vi "test_SetItemInfoDependencies.vi"() -> (3 "Pass?":bool)   [LabVIEW 2020, in "Tests.SolutionBuilder.lvlib"]
uses:
  Tests.SolutionBuilder.lvlib
  SolutionBuilder/SolutionBuilder.lvclass
  SolutionBuilder/ProjectItem/ProjectItem.lvclass
panel:
  out "test results":u32 format="%02b"
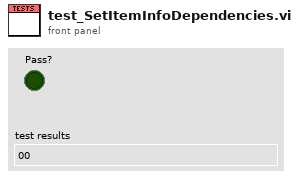
[diagram p1: front panel]
types:
  T1 = cluster{"Relative Path from 1 to 2":path, string[]}[]
  T2 = typedef "SolutionBuilder.lvlib/SolutionBuilder.lvclass/ProjectItemMap.ctl" = map{path, refnum<class "ProjectItem.lvclass">[]}
  T3 = cluster{"Relative Path from 1 to 2":path, string[]}
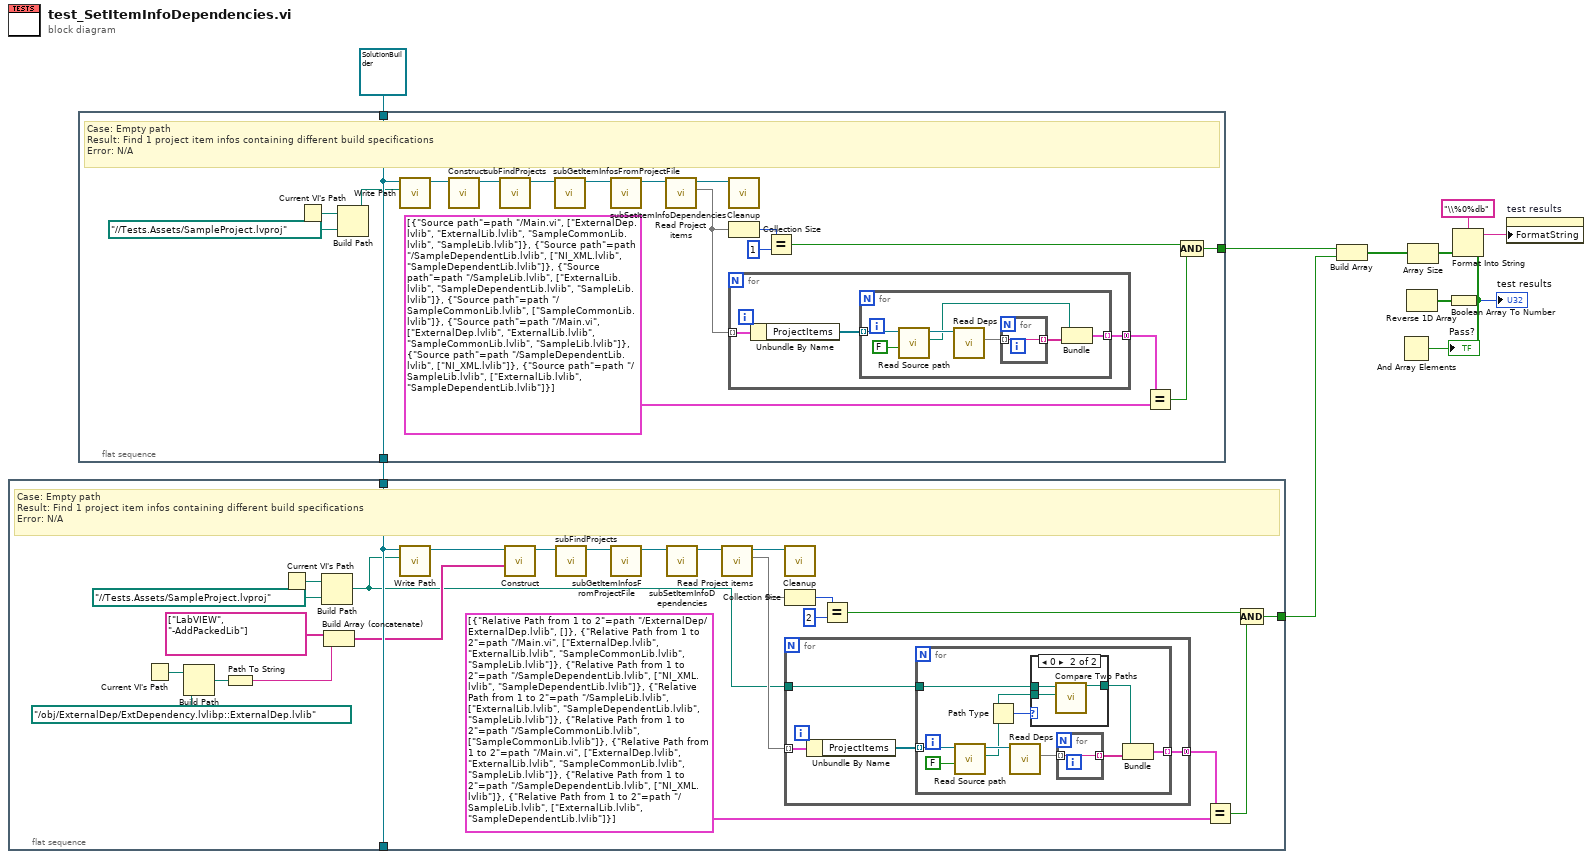
[diagram p0: block diagram]
diagram:
  n1 = flat-sequence {
    tunnel: [w27] -> w1
    tunnel: w2 -> [w35]
    tunnel: [w35] -> _
    frame #0 {
      # "Case: Empty path\nResult: Find 1 project item infos containing different build specifications\nError: N/A"
      n2 = Current VI's Path() -> (path=w16:path)
      n3 = Build Path(base path=w16, name or relative path=path "../obj/ExternalDep/ExtDependency.lvlibp::ExternalDep.lvlib" ("Path")) -> (appended path=w18:path)
      n4 = Path To String(path=w18) -> (string=w19:string)
      n5 = Current VI's Path() -> (path=w33:path)
      n6 = Build Path(base path=w33, name or relative path=path "../../Tests.Assets/SampleProject.lvproj" ("Path")) -> (appended path=w13:path)
      n7 = Build Array (concatenate)(string[] ["LabVIEW", "-AddPackedLib"] ("App.Args"), w19) -> (w17:string[])
      n8 = call-dynamic "Write Path.vi"("Path"=w13, "SolutionBuilder in"=w35) -> ("SolutionBuilder out"=w24:refnum<class "SolutionBuilder.lvclass">)  [unwired: 9 in]
      n9 = call-dynamic "Construct.vi"("App.Args"=w17, "SolutionBuilder in"=w24) -> ("SolutionBuilder out"=w23:refnum<class "SolutionBuilder.lvclass">)  [unwired: 8 in, 1 out]
      n10 = call "subFindProjects.vi"("SolutionBuilder in"=w23) -> ("SolutionBuilder out"=w34:refnum<class "SolutionBuilder.lvclass">)  [unwired: 9 in, 1 out]
      n11 = call "subGetItemInfosFromProjectFile.vi"("SolutionBuilder in"=w34) -> ("SolutionBuilder out"=w26:refnum<class "SolutionBuilder.lvclass">)  [unwired: 9 in, 1 out]
      n12 = call "subSetItemInfoDependencies.vi"("SolutionBuilder in"=w26) -> ("SolutionBuilder out"=w25:refnum<class "SolutionBuilder.lvclass">)  [unwired: 9 in, 1 out]
      n13 = call-dynamic "Read Project items.vi"("SolutionBuilder in"=w25) -> ("Project items"=w29:T2, "SolutionBuilder out"=w22:refnum<class "SolutionBuilder.lvclass">)  [unwired: 9 in]
      n14 = call-dynamic "Cleanup.vi"("SolutionBuilder in"=w22) -> ()  [unwired: 9 in, 2 out]
      n15 = Collection Size(1:w29) -> (0:w31:i32)
      n16 = for {
        tunnel: w29 -> [w39] mode=indexing
        tunnel: [w37] -> w14 mode=concatenating
        tunnel: w13 -> [w36]
        n17 = Unbundle By Name(w39) -> ("ProjectItems"=w38:refnum<class "ProjectItem.lvclass">[])
        n18 = for {
          tunnel: w38 -> [w46] mode=indexing
          tunnel: [w47] -> w37 mode=indexing
          tunnel: w36 -> [w40]
          n19 = call-dynamic "Read Source path.vi"("Force abs path? (T)"=FALSE, "ProjectItem in"=w46) -> ("Source path"=w42:path, "ProjectItem out"=w45:refnum<class "ProjectItem.lvclass">)  [unwired: 8 in]
          n20 = Path Type(1:w42) -> (0:w43:i16)
          n21 = call-dynamic "Read Deps.vi"("ProjectItem in"=w45) -> ("Deps"=w49:set{string})  [unwired: 9 in, 1 out]
          n22 = case shown="0" w43 {
            tunnel: w42 -> [w50 w51]
            tunnel: [w50 w53] -> w41
            tunnel: w40 -> [_ w52]
            frame Default {
            }
            frame 0 {
              n23 = call <vilib>:"Compare Two Paths.vi"("Path 2"=w51, "Path 1"=w52) -> ("Relative Path from 1 to 2"=w53:path)  [unwired: 6 in, 3 out]
            }
          }
          n24 = for {
            tunnel: w49 -> [w54] mode=indexing
            tunnel: [w54] -> w48 mode=indexing
          }
          n25 = Bundle("Relative Path from 1 to 2"=w41, w48) -> (w47:T3)  [unwired: 1 in]
        }
      }
      n26 = Equal?(x=w31, y=2) -> (x = y?=w28:bool)
      n27 = Equal?(x=w14, y=T1 [{"Relative Path from 1 to 2"=path "../ExternalDep/ExternalDep.lvlib", []}, {"Relative Path from 1 to 2"=path "../Main.vi", ["ExternalDep.lvlib", "ExternalLib.lvlib", "SampleCommonLib.lvlib", "SampleLib.lvlib"]}, {"Relative Path from 1 to 2"=path "../SampleDependentLib.lvlib", ["NI_XML.lvlib", "SampleDependentLib.lvlib"]}, {"Relative Path from 1 to 2"=path "../SampleLib.lvlib", ["ExternalLib.lvlib", "SampleDependentLib.lvlib", "SampleLib.lvlib"]}, {"Relative Path from 1 to 2"=path "../SampleCommonLib.lvlib", ["SampleCommonLib.lvlib"]}, {"Relative Path from 1 to 2"=path "../Main.vi", ["ExternalDep.lvlib", "ExternalLib.lvlib", "SampleCommonLib.lvlib", "SampleLib.lvlib"]}, {"Relative Path from 1 to 2"=path "../SampleDependentLib.lvlib", ["NI_XML.lvlib"]}, {"Relative Path from 1 to 2"=path "../SampleLib.lvlib", ["ExternalLib.lvlib", "SampleDependentLib.lvlib"]}] ("Array 2")) -> (x = y?=w21:bool)
      n28 = Compound Arithmetic op=AND(w28, w21) -> (w27:bool)
    }
  }
  n29 = flat-sequence {
    tunnel: [w63] -> w5
    tunnel: refnum<class "SolutionBuilder.lvclass"> refnum ("SolutionBuilder in") -> [w72]
    tunnel: [w72] -> w2
    frame #0 {
      # "Case: Empty path\nResult: Find 1 project item infos containing different build specifications\nError: N/A"
      n30 = Current VI's Path() -> (path=w70:path)
      n31 = Build Path(base path=w70, name or relative path=path "../../Tests.Assets/SampleProject.lvproj" ("Path")) -> (appended path=w68:path)
      n32 = call-dynamic "Write Path.vi"("Path"=w68, "SolutionBuilder in"=w72) -> ("SolutionBuilder out"=w60:refnum<class "SolutionBuilder.lvclass">)  [unwired: 9 in]
      n33 = call-dynamic "Construct.vi"("SolutionBuilder in"=w60) -> ("SolutionBuilder out"=w59:refnum<class "SolutionBuilder.lvclass">)  [unwired: 9 in, 1 out]
      n34 = call "subFindProjects.vi"("SolutionBuilder in"=w59) -> ("SolutionBuilder out"=w71:refnum<class "SolutionBuilder.lvclass">)  [unwired: 9 in, 1 out]
      n35 = call "subGetItemInfosFromProjectFile.vi"("SolutionBuilder in"=w71) -> ("SolutionBuilder out"=w62:refnum<class "SolutionBuilder.lvclass">)  [unwired: 9 in, 1 out]
      n36 = call "subSetItemInfoDependencies.vi"("SolutionBuilder in"=w62) -> ("SolutionBuilder out"=w61:refnum<class "SolutionBuilder.lvclass">)  [unwired: 9 in, 1 out]
      n37 = call-dynamic "Read Project items.vi"("SolutionBuilder in"=w61) -> ("Project items"=w65:T2, "SolutionBuilder out"=w57:refnum<class "SolutionBuilder.lvclass">)  [unwired: 9 in]
      n38 = call-dynamic "Cleanup.vi"("SolutionBuilder in"=w57) -> ()  [unwired: 9 in, 2 out]
      n39 = Collection Size(1:w65) -> (0:w67:i32)
      n40 = for {
        tunnel: w65 -> [w75] mode=indexing
        tunnel: [w73] -> w56 mode=concatenating
        n41 = Unbundle By Name(w75) -> ("ProjectItems"=w74:refnum<class "ProjectItem.lvclass">[])
        n42 = for {
          tunnel: w74 -> [w79] mode=indexing
          tunnel: [w80] -> w73 mode=indexing
          n43 = call-dynamic "Read Source path.vi"("Force abs path? (T)"=FALSE, "ProjectItem in"=w79) -> ("Source path"=w77:path, "ProjectItem out"=w78:refnum<class "ProjectItem.lvclass">)  [unwired: 8 in]
          n44 = call-dynamic "Read Deps.vi"("ProjectItem in"=w78) -> ("Deps"=w82:set{string})  [unwired: 9 in, 1 out]
          n45 = for {
            tunnel: w82 -> [w83] mode=indexing
            tunnel: [w83] -> w81 mode=indexing
          }
          n46 = Bundle("Source path"=w77, w81) -> (w80:cluster{"Source path":path, string[]})  [unwired: 1 in]
        }
      }
      n47 = Equal?(x=w67, y=1) -> (x = y?=w64:bool)
      n48 = Equal?(x=w56, y=cluster{"Source path":path, string[]}[] [{"Source path"=path "../Main.vi", ["ExternalDep.lvlib", "ExternalLib.lvlib", "SampleCommonLib.lvlib", "SampleLib.lvlib"]}, {"Source path"=path "../SampleDependentLib.lvlib", ["NI_XML.lvlib", "SampleDependentLib.lvlib"]}, {"Source path"=path "../SampleLib.lvlib", ["ExternalLib.lvlib", "SampleDependentLib.lvlib", "SampleLib.lvlib"]}, {"Source path"=path "../SampleCommonLib.lvlib", ["SampleCommonLib.lvlib"]}, {"Source path"=path "../Main.vi", ["ExternalDep.lvlib", "ExternalLib.lvlib", "SampleCommonLib.lvlib", "SampleLib.lvlib"]}, {"Source path"=path "../SampleDependentLib.lvlib", ["NI_XML.lvlib"]}, {"Source path"=path "../SampleLib.lvlib", ["ExternalLib.lvlib", "SampleDependentLib.lvlib"]}] ("Array")) -> (x = y?=w58:bool)
      n49 = Compound Arithmetic op=AND(w64, w58) -> (w63:bool)
    }
  }
  n50 = Build Array(w5, w1) -> (w9:bool[])
  n51 = And Array Elements(Boolean array=w9) -> (logical AND=→"Pass?":bool)
  n52 = Reverse 1D Array(array=w9) -> (reversed array=w4:bool[])
  n53 = Array Size(array=w9) -> (size(s)=w7:i32)
  n54 = Boolean Array To Number(Boolean array=w4) -> (number=→"test results":u32)
  n55 = Format Into String(format string="\\%0%db", w7) -> (resulting string=w6:string)  [unwired: 2 in, 1 out]
  n56 = property on="test results" class="DigNum (strict)"("FormatString"=w6) -> ()  [unwired: 2 in, 2 out]
